vi "Update Motor Speed Settings.vi"(8 "error in (no error)":errorcluster, 10 "Motor_Speed Setting Ref Array":refnum<vi>[](array[refnum]), 11 "Bool RefIn":refnum<vi>) -> (0 "error out":errorcluster, 3 "Motor Speed":dbl)   [LabVIEW 2018]
uses:
  <vilib>/Utility/miscctls.llb/LVTextColorsTypeDef.ctl
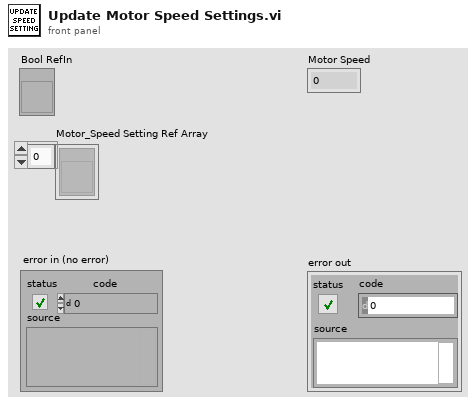
[diagram p1: front panel]
types:
  T1 = enum8{"Enabled", "Disabled", "Disabled and Grayed Out"}
  T2 = typedef "LVTextColorsTypeDef.ctl" = cluster{"Text Color":u32, "Background Color":u32}
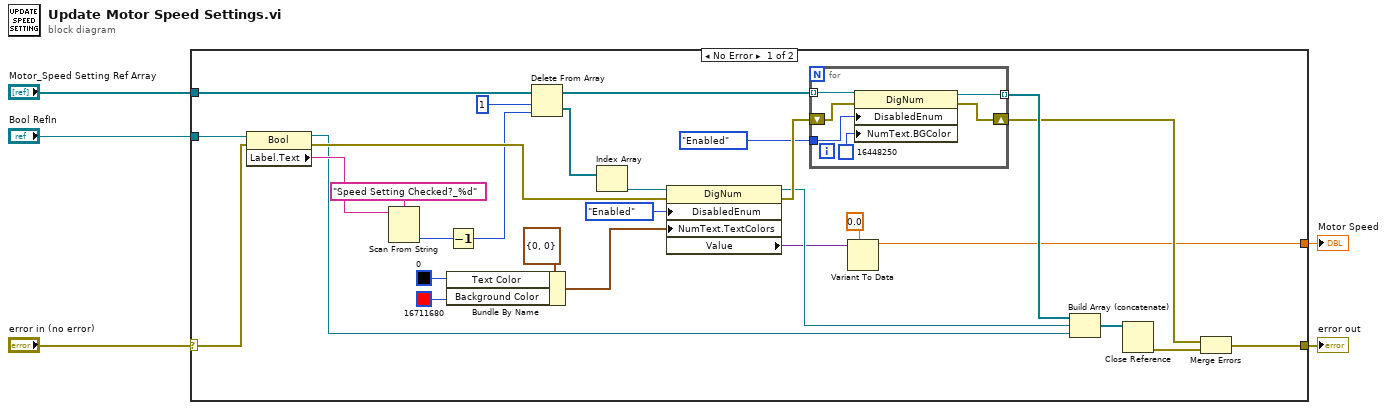
[diagram p0: block diagram]
diagram:
  n1 = case shown="No Error" "error in (no error)" {
    selector: "error in (no error)" -> [w33 w41]
    tunnel: "Bool RefIn" -> [w34 _]
    tunnel: "Motor_Speed Setting Ref Array" -> [w29 _]
    tunnel: [w9 w41] -> w2
    tunnel: [w6 _] -> w1
    frame No Error {
      n2 = property class="Bool"(reference=w34, error in=w33) -> (reference out=w15:refnum<vi>, error out=w30:errorcluster, "Label.Text"=w32:string)
      n3 = Scan From String(format string="Speed Setting Checked?_%d", input string=w32) -> (output 1=w27:i32)  [unwired: 3 in, 3 out]
      n4 = Bundle By Name(cluster=T2 {"Text Color"=0, "Background Color"=0} ("Numeric Text.Text Colors"), "Text Color"=u32 0, "Background Color"=u32 16711680) -> (w19:T2)
      n5 = Decrement(x=w27) -> (x-1=w26:i32)
      n6 = Delete From Array(array=w29, length=1, index=w26) -> (deleted portion=w25:refnum<vi>[], array with subset deleted=w18:refnum<vi>[])
      n7 = Index Array(array=w25) -> (element=w24:refnum<vi>)  [unwired: 1 in]
      n8 = property class="DigNum"(reference=w24, error in=w30, "DisabledEnum"=T1."Enabled" ("Disabled"), "NumText.TextColors"=w19) -> (reference out=w14:refnum<vi>, error out=w17:errorcluster, "Value"=w8:variant)
      n9 = for {
        tunnel: w18 -> [w40] mode=indexing
        shift-right: [w37] -> w11
        shift-left: w17 -> [w38]
        tunnel: [w39] -> w13 mode=indexing
        tunnel: T1."Enabled" ("Disabled") -> [w36]
        n10 = property class="DigNum"(reference=w40, error in=w38, "DisabledEnum"=w36, "NumText.BGColor"=u32 16448250) -> (reference out=w39:refnum<vi>, error out=w37:errorcluster)
      }
      n11 = Variant To Data(type=0.0, Variant=w8) -> (data=w6:dbl)  [unwired: 1 in, 1 out]
      n12 = Build Array (concatenate)(w13, w14, w15) -> (w12:refnum<vi>[])
      n13 = Close Reference(reference=w12) -> (error out=w10:errorcluster)  [unwired: 1 in]
      n14 = Merge Errors(w11, w10) -> (w9:errorcluster)
    }
    frame Error {
    }
  }
  "error out" <- w2
  "Motor Speed" <- w1
